vi "SetMenuItems.vi"(8 "error in (no error)":errorcluster, 10 "Menu Items":refnum<data-value>[](array[refnum]), 11 "MGI_Menu in":refnum<class "MGI_Menu.lvclass">) -> (0 "error out":errorcluster, 3 "MGI_Menu out":refnum<class "MGI_Menu.lvclass">)   [LabVIEW 2016, in "MGI_Menu.lvclass"]
doc: "Authored by Derek E. Trepanier\nsupport@mooregoodideas.com\nwww.mooregoodideas.com\n\nCopyright (c) 2012, Moore Good Ideas, Inc.\n\nAll rights reserved.\n\nRedistribution and use in source and binary forms, with or without modification, are permitted provided that the following conditions are met:\n\n * Redistributions of source code must retain the above copyright notice, this list of conditions and the following disclaimer.\n * Redistributions in binary form must reproduce the above copyright notice, this list of conditions and the following disclaimer in the documentation and/or other materials provided with the distribution.\n * Neither the name of Moore Good Ideas, Inc. nor the names of its contributors may be used to endorse or promote products derived from this software without specific prior written permission.\n\nTHIS SOFTWARE IS PROVIDED BY THE COPYRIGHT HOLDERS AND CONTRIBUTORS \"AS IS\" AND ANY EXPRESS OR IMPLIED WARRANTIES, INCLUDING, BUT NOT LIMITED TO, THE IMPLIED WARRANTIES OF MERCHANTABILITY AND FITNESS FOR A PARTICULAR PURPOSE ARE DISCLAIMED. IN NO EVENT SHALL THE COPYRIGHT OWNER OR CONTRIBUTORS BE LIABLE FOR ANY DIRECT, INDIRECT, INCIDENTAL, SPECIAL, EXEMPLARY, OR CONSEQUENTIAL DAMAGES (INCLUDING, BUT NOT LIMITED TO, PROCUREMENT OF SUBSTITUTE GOODS OR SERVICES; LOSS OF USE, DATA, OR PROFITS; OR BUSINESS INTERRUPTION) HOWEVER CAUSED AND ON ANY THEORY OF LIABILITY, WHETHER IN CONTRACT, STRICT LIABILITY, OR TORT (INCLUDING NEGLIGENCE OR OTHERWISE) ARISING IN ANY WAY OUT OF THE USE OF THIS SOFTWARE, EVEN IF ADVISED OF THE POSSIBILITY OF SUCH DAMAGE."
uses:
  <userlib>/_MGI/Menu Building/MenuTypes/MGI_Menu.lvclass
  <userlib>/_MGI/Menu Building/MenuItem/MGI_MenuItem.lvclass
  <userlib>/_MGI/Menu Building/MenuTypes/MGI_Menu.lvclass/MGI_Menu.ctl
  <userlib>/_MGI/Menu Building/MenuItem/Read Tag.vi
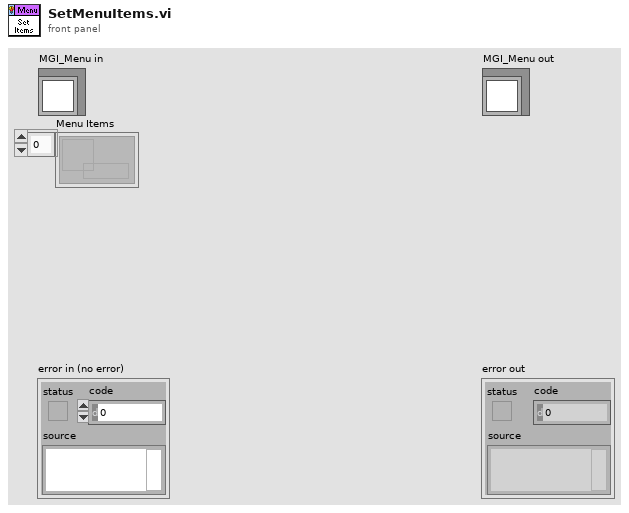
[diagram p1: front panel]
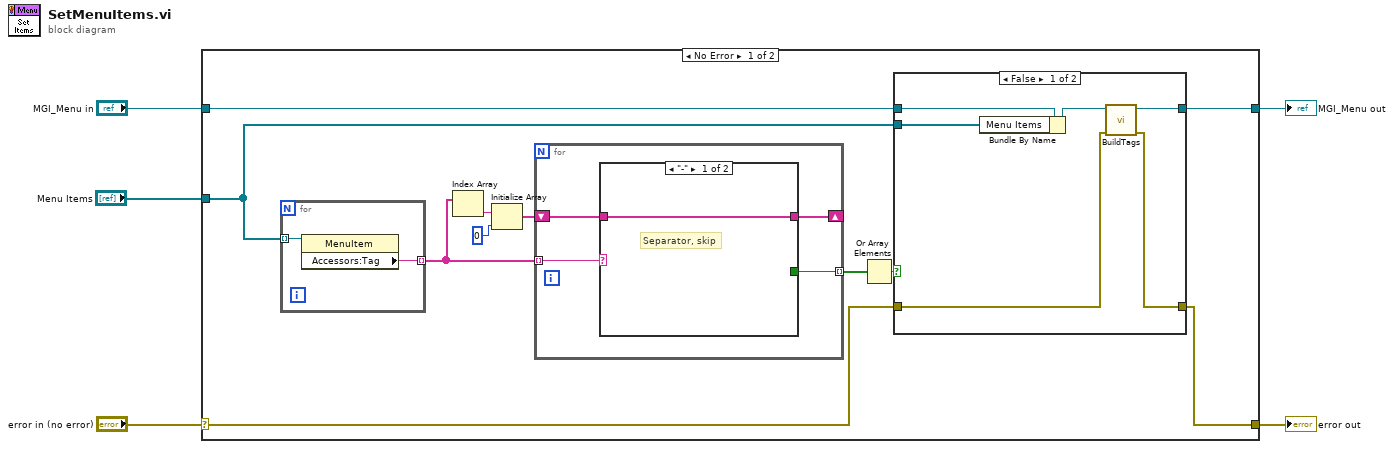
[diagram p0: block diagram]
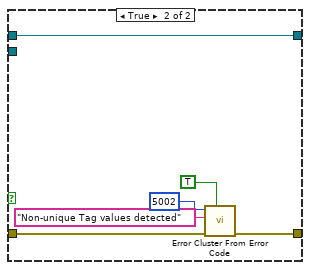
[diagram p2: hidden frame]
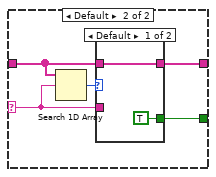
[diagram p3: hidden frame]
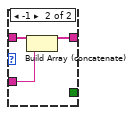
[diagram p4: hidden frame]
diagram:
  n1 = case shown="No Error" "error in (no error)" {
    selector: "error in (no error)" -> [w10 w47]
    tunnel: [w9 w47] -> w4
    tunnel: [w6 w46] -> w2
    tunnel: "MGI_Menu in" -> [w8 w46]
    tunnel: "Menu Items" -> [w7 _]
    frame No Error {
      n2 = for {
        tunnel: w7 -> [w45] mode=indexing
        tunnel: [w44] -> w13 mode=indexing
        n3 = property class="MenuItem"(reference=w45) -> ("Accessors:Tag"=w44:string)  [unwired: 1 in, 2 out]
      }
      n4 = Index Array(array=w13) -> (element=w16:string)  [unwired: 1 in]
      n5 = Initialize Array(w16, 0 ("Dimension Size")) -> (w15:string[])
      n6 = for {
        tunnel: w13 -> [w29] mode=indexing
        shift-right: [w32] -> _
        shift-left: w15 -> [w31]
        tunnel: [w30] -> w12 mode=indexing
        n7 = case shown="\"-\"" w29 {
          selector: w29 -> [_ w34]
          tunnel: [w33 w37] -> w32
          tunnel: w31 -> [w33 w36]
          tunnel: [_ w35] -> w30
          frame "-" {
            # "Separator, skip"
          }
          frame Default {
            n8 = Search 1D Array(1D array=w36, element=w34) -> (index of element=w38:i32)  [unwired: 1 in]
            n9 = case shown="Default" w38 {
              tunnel: w34 -> [_ w43]
              tunnel: [w40 w41] -> w37
              tunnel: w36 -> [w40 w42]
              tunnel: [TRUE _] -> w35
              frame Default {
              }
              frame -1 {
                n10 = Build Array (concatenate)(w42, w43) -> (w41:string[])
              }
            }
          }
        }
      }
      n11 = Or Array Elements(Boolean array=w12) -> (logical OR=w11:bool)
      n12 = case shown="False" w11 {
        tunnel: w10 -> [w18 w28]
        tunnel: [w17 w27] -> w9
        tunnel: [w19 w23] -> w6
        tunnel: w8 -> [w22 w23]
        tunnel: w7 -> [w21 _]
        frame False {
          n13 = Bundle By Name(cluster=w22, "Menu Items"=w21) -> (w20:refnum<class "MGI_Menu.lvclass">)
          n14 = call <userlib>:"BuildTags.vi"("error in (no error)"=w18, "Menu in"=w20) -> ("error out"=w17:errorcluster, "Menu out"=w19:refnum<class "MGI_Menu.lvclass">)  [unwired: 8 in]
        }
        frame True {
          n15 = call <vilib>:"Error Cluster From Error Code.vi"("show call chain? (False)"=TRUE, "error in (no error)"=w28, "error message (\"\")"="Non-unique Tag values detected" ("error message (\"\")"), "error code (0)"=5002) -> ("error out"=w27:errorcluster)  [unwired: 5 in]
        }
      }
    }
    frame Error {
    }
  }
  "error out" <- w4
  "MGI_Menu out" <- w2
